vi "MultiplyDivide.vi"() -> ()   [LabVIEW 2015]
panel:
  out "Result":dbl
  in  "?":bool
  in  "Y":dbl
  in  "X":dbl
  # "Multiply XY -(T)"
  # "Divide X/Y (F)"
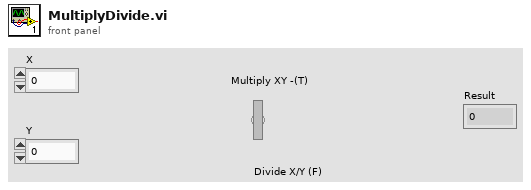
[diagram p1: front panel]
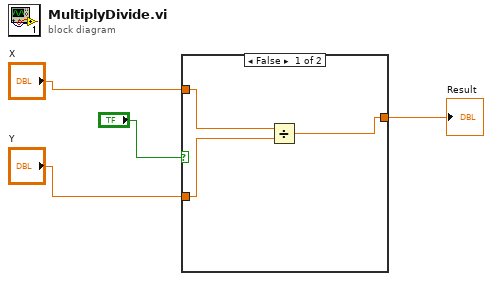
[diagram p0: block diagram]
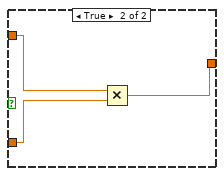
[diagram p2: hidden frame]
diagram:
  n1 = case shown="False" "?" {
    tunnel: "X" -> [w7 w9]
    tunnel: "Y" -> [w6 w10]
    tunnel: [w5 w8] -> w1
    frame False {
      n2 = Divide(x=w7, y=w6) -> (x/y=w5:dbl)
    }
    frame True {
      n3 = Multiply(x=w9, y=w10) -> (x*y=w8:dbl)
    }
  }
  "Result" <- w1
